vi "Initialize Game.vi"(10 "Height":u32, 11 "Width":u32) -> (3 "Array":bool[][](array[boolean]))   [LabVIEW 2021, in "Game of Life.lvlib"]
doc: "This VI generates a 2D boolean array of living cells in a random fashion with 30% living cell rate."
uses:
  Game of Life.lvlib
  <vilib>/numeric/Random Number (Range) U64.vi
  <vilib>/numeric/sub_Random U32.vi
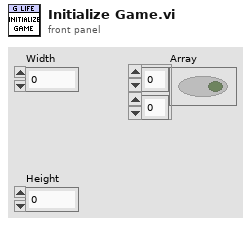
[diagram p1: front panel]
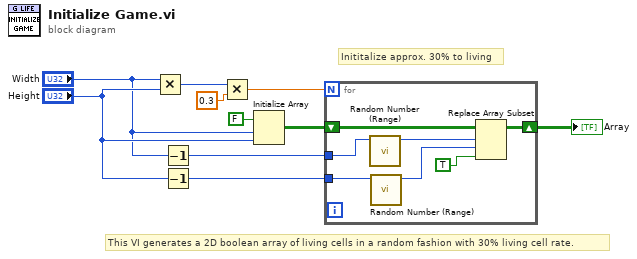
[diagram p0: block diagram]
diagram:
  # "This VI generates a 2D boolean array of living cells in a random fashion with 30% living cell rate."
  # "Inititalize approx. 30% to living"
  n1 = Multiply(x="Width", y="Height") -> (x*y=w5:u32)
  n2 = Decrement(x="Width") -> (x-1=w2:u32)
  n3 = Decrement(x="Height") -> (x-1=w3:u32)
  n4 = Multiply(x=w5, y=0.3) -> (x*y=w7:dbl)
  n5 = Initialize Array(FALSE, "Width", "Height") -> (w4:bool[][])
  n6 = for {
    N: w7 -> [_]
    tunnel: w2 -> [w17]
    tunnel: w3 -> [w16]
    shift-right: [w11] -> w8
    shift-left: w4 -> [w15]
    n7 = call-poly <vilib>:"Random Number (Range).vi"("upper bound (100)"=w17) -> ("number"=w14:u64)  [unwired: 10 in]
    n8 = call-poly <vilib>:"Random Number (Range).vi"("upper bound (100)"=w16) -> ("number"=w13:u64)  [unwired: 10 in]
    n9 = Replace Array Subset(array=w15, new element=TRUE ("new element/subarray"), index (row)=w14, index (col)=w13) -> (w11:bool[][])
  }
  "Array" <- w8
